vi "FdxCmdTxCreateHiResVLCvi.vi"(8 "error in":errorcluster, 9 "TransmitVLHiRes":T1 {"NetSelect" items=["FDX_TX_FRAME_DLY_A"=0, "FDX_TX_FRAME_DLY_B"=1, "FDX_TX_FRAME_BOTH "=3, "FDX_TX_FRAME_ONLY_A"=4, "FDX_TX_FRAME_ONLY_B "=5]}, 11 "InstrumentHandle_port":u32) -> (0 "error out":errorcluster, 3 "InstrumentHandle_port":u32)   [LabVIEW 2020, in "AIM664LV.lvlib"]
doc: "This function is used to setup a Virtual Link to transmit data. This is only a description of the\nVirtual Link specific parameters, which must be known by the system for transmitting. This\nfunction can be used only when the transmitter is not running. This function is used to specify a\nVL with a high resolution bag."
uses:
  AIM664LV.lvlib
  AFDX_LibraryAdmin/FdxGlobalDllPath.vi
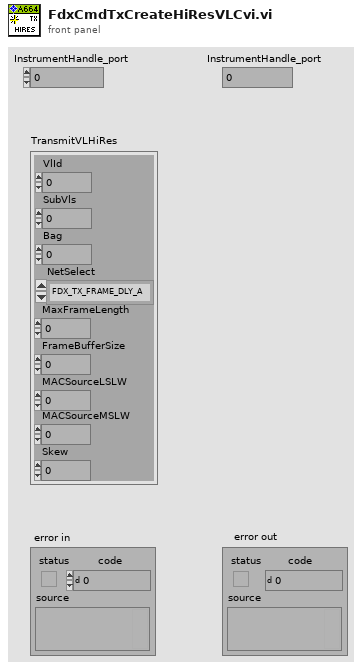
[diagram p1: front panel]
types:
  T1 = cluster{"VlId":u32, "SubVls":u32, "Bag":u32, "NetSelect":u32, "MaxFrameLength":u32, "FrameBufferSize":u32, "MACSourceLSLW":u32, "MACSourceMSLW":u32, "Skew":u32}
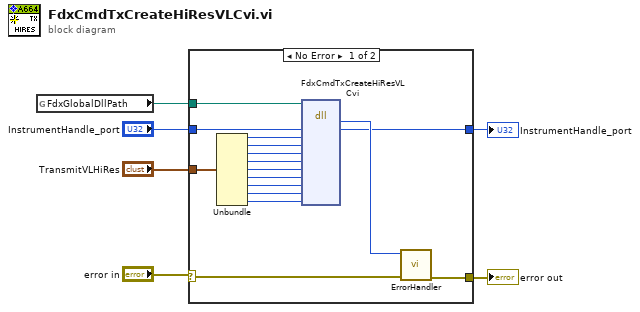
[diagram p0: block diagram]
diagram:
  n1 = global read "FdxGlobalDllPath.vi" "FdxGlobalDllPath"() -> (w4:path)
  n2 = case shown="No Error" "error in" {
    selector: "error in" -> [w21 w24]
    tunnel: [w22 w24] -> w6
    tunnel: w4 -> [w10 _]
    tunnel: "InstrumentHandle_port" -> [w9 w23]
    tunnel: [w8 w23] -> w2
    tunnel: "TransmitVLHiRes" -> [w7 _]
    frame No Error {
      n3 = Unbundle(w7) -> ("VlId"=w19:u32, "SubVls"=w18:u32, "Bag"=w17:u32, "NetSelect"=w16:u32, "MaxFrameLength"=w15:u32, "FrameBufferSize"=w14:u32, "MACSourceLSLW"=w13:u32, "MACSourceMSLW"=w12:u32, "Skew"=w11:u32)
      n4 = dll-call lib="aim_fdx.19.dll" fn="FdxCmdTxCreateHiResVLCvi"(path in=w10, "InstrumentHandle"=w9, "VlId"=w19, "SubVls"=w18, "Bag"=w17, "NetSelect"=w16, "MaxFrameLength"=w15, "FrameBufferSize"=w14, "MACSourceLSLW"=w13, "MACSourceMSLW"=w12, "Skew"=w11) -> ("status"=w20:i32, "InstrumentHandle"=w8:u32)  [unwired: 11 in, 2 out]
      n5 = call "ErrorHandler.vi"("error in"=w21, "AIM Error"=w20) -> ("error out"=w22:errorcluster)  [unwired: 9 in]
    }
    frame Error {
    }
  }
  "error out" <- w6
  "InstrumentHandle_port" <- w2
